vi "TDMS_Save_to_CSV.vi"() -> ()   [LabVIEW 2018]
uses:
  <vilib>/Utility/file.llb/Write Delimited Spreadsheet (I64).vi
panel:
  out "error out":errorcluster
  out "size(s) 2":i32[](array[numeric])
  out "size(s)":i32[](array[numeric])
  out "Data out":i32[][](array[numeric])
  in  "CSV file to save":path=path "D:/Users_Data/Dmitriy_T/Documents/F5/Design & Development/Lick sensor/Capsensor_6-17-2020_10.56 AM_072cee.csv"
  out "Timestamp":string[](array[string])
  in  "TDMS file to open":path=path "D:/Users_Data/Dmitriy_T/Documents/F5/Design & Development/Lick sensor/Capsensor_6-17-2020_10.56 AM_072cee.tdms"
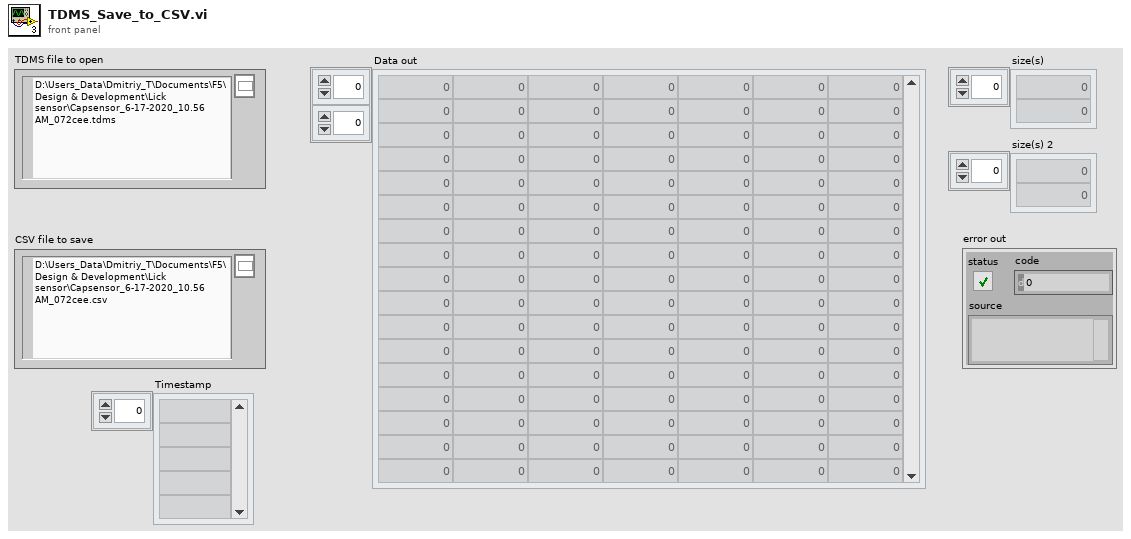
[diagram p1: front panel]
types:
  T1 = enum16{"open", "open or create", "create or replace", "create", "open (read-only)"}
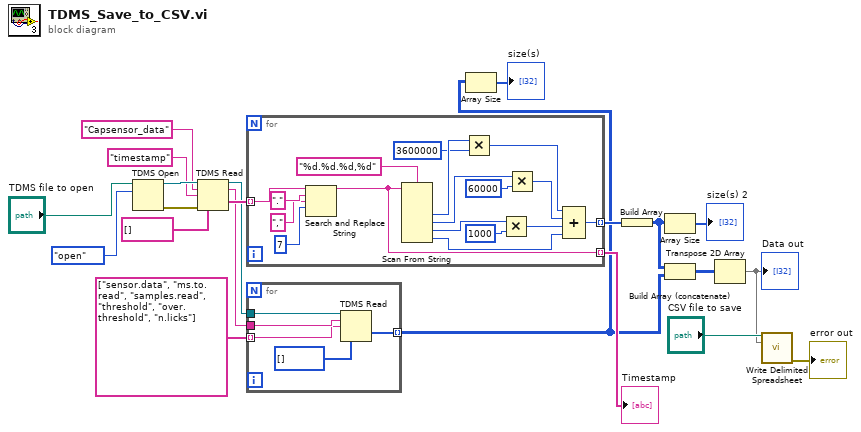
[diagram p0: block diagram]
diagram:
  n1 = TDMS Open(10:T1."open" ("operation (0:open)"), 11:"TDMS file to open") -> (0:w20:errorcluster, 3:w19:refnum<k34>)  [unwired: 5 in]
  n2 = TDMS Read(0:w19, 5:"Capsensor_data" ("group name in"), 7:"timestamp" ("group name in"), 11:w20, 12:string[] []) -> (4:w13:refnum<k34>, 6:w12:string, 10:w15:string[])  [unwired: 3 in, 3 out]
  n3 = for {
    tunnel: w15 -> [w38] mode=indexing
    tunnel: [w34] -> w14 mode=indexing
    tunnel: [w26] -> w8 mode=indexing
    n4 = Search and Replace String(input string=w38, search string=".", replace string="," ("replace string (\"\")"), offset=7 ("offset (0)")) -> (result string=w34:string)  [unwired: 4 in, 3 out]
    n5 = Scan From String(format string="%d.%d.%d,%d", input string=w34) -> (output 1=w32:i32, output 2=w31:i32, output 3=w24:i32, output 4=w22:i32)  [unwired: 6 in, 3 out]
    n6 = Multiply(x=w32, y=3600000) -> (x*y=w28:i32)
    n7 = Multiply(x=w24, y=1000) -> (x*y=w23:i32)
    n8 = Multiply(x=w31, y=60000) -> (x*y=w27:i32)
    n9 = Compound Arithmetic op=ADD(w28, w27, w23, w22) -> (w26:i32)
  }
  "Timestamp" <- w14
  n10 = for {
    tunnel: w13 -> [w43]
    tunnel: w12 -> [w42]
    tunnel: string[] ["sensor.data", "ms.to.read", "samples.read", "threshold", "over.threshold", "n.licks"] -> [w41] mode=indexing
    tunnel: [w40] -> w3 mode=indexing
    n11 = TDMS Read(0:w43, 5:w42, 7:w41, 12:i32[] []) -> (10:w40:i32[])  [unwired: 4 in, 5 out]
  }
  n12 = Array Size(array=w3) -> (size(s)=→"size(s)":i32[])
  n13 = Build Array(w8) -> (w4:i32[][])
  n14 = Array Size(array=w4) -> (size(s)=→"size(s) 2":i32[])
  n15 = Build Array (concatenate)(w4, w3) -> (w7:i32[][])
  n16 = Transpose 2D Array(2D array=w7) -> (transposed array=w2:i32[][])
  "Data out" <- w2
  n17 = call-poly <vilib>:"Write Delimited Spreadsheet.vi"("file path (dialog if empty)"="CSV file to save", "2D data"=w2) -> ("error out"=→"error out":errorcluster)  [unwired: 12 in, 1 out]
